vi "Evaluate ECU ID String.vi"(1 "String In":string) -> (0 "Test OK":bool)   [LabVIEW 2023]
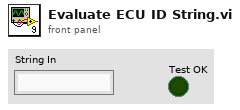
[diagram p1: front panel]
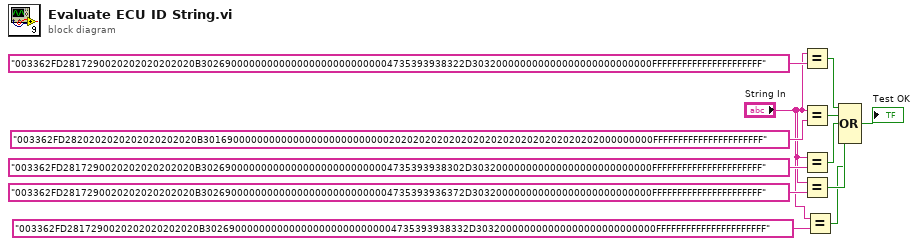
[diagram p0: block diagram]
diagram:
  n1 = Equal?(x="String In", y="003362FD2817290020202020202020B30269000000000000000000000000004735393938322D303200000000000000000000000000FFFFFFFFFFFFFFFFFFFFFF") -> (x = y?=w9:bool)
  n2 = Equal?(x="String In", y="003362FD2820202020202020202020B301690000000000000000000000000020202020202020202020202020202020202000000000FFFFFFFFFFFFFFFFFFFFFF") -> (x = y?=w8:bool)
  n3 = Equal?(x="String In", y="003362FD2817290020202020202020B30269000000000000000000000000004735393938302D303200000000000000000000000000FFFFFFFFFFFFFFFFFFFFFF") -> (x = y?=w7:bool)
  n4 = Equal?(x="String In", y="003362FD2817290020202020202020B30269000000000000000000000000004735393936372D303200000000000000000000000000FFFFFFFFFFFFFFFFFFFFFF") -> (x = y?=w4:bool)
  n5 = Equal?(x="String In", y="003362FD2817290020202020202020B30269000000000000000000000000004735393938332D303200000000000000000000000000FFFFFFFFFFFFFFFFFFFFFF") -> (x = y?=w1:bool)
  n6 = Compound Arithmetic op=OR(w9, w8, w7, w4, w1) -> (→"Test OK":bool)
